vi "Init Request Poller.vi"(8 "error in (no error)":errorcluster, 10 "output_request_poller in":refnum<class "output_poller.lvclass">, 11 "output in":refnum<class "Output.lvclass">) -> (0 "error out":errorcluster, 3 "output out":refnum<class "Output.lvclass">)   [LabVIEW 2015, in "Output.lvclass"]
uses:
  Output.lvclass
  output_poller/output_poller.lvclass
  Output.lvclass/Output.ctl
  output_poller/output_poller.lvclass/output_poller.ctl
  <vilib>/ActorFramework/Actor/Actor.lvclass
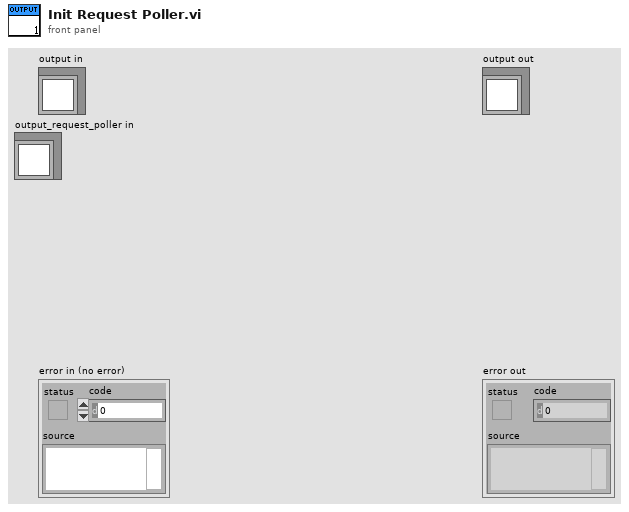
[diagram p1: front panel]
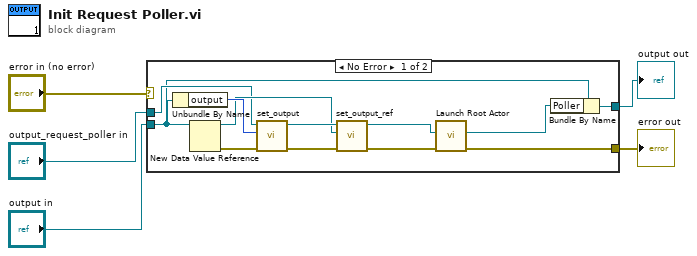
[diagram p0: block diagram]
diagram:
  n1 = case shown="No Error" "error in (no error)" {
    selector: "error in (no error)" -> [_ w19]
    tunnel: [w10 w19] -> w4
    tunnel: [w6 w18] -> w2
    tunnel: "output in" -> [w7 w18]
    tunnel: "output_request_poller in" -> [w9 _]
    frame No Error {
      n2 = Unbundle By Name(w7) -> ("output"=w16:i32)
      n3 = New Data Value Reference(data value=w7) -> (data value reference=w15:refnum<data-value>, error out=w13:errorcluster)  [unwired: 1 in]
      n4 = call "set_output.vi"("error in (no error)"=w13, "output"=w16, "output_request_poller in"=w9) -> ("error out"=w12:errorcluster, "output_request_poller out"=w17:refnum<class "output_poller.lvclass">)  [unwired: 7 in]
      n5 = call "set_output_ref.vi"("error in (no error)"=w12, "output_ref"=w15, "output_request_poller in"=w17) -> ("error out"=w11:errorcluster, "output_request_poller out"=w14:refnum<class "output_poller.lvclass">)  [unwired: 7 in]
      n6 = call <vilib>:"Launch Root Actor.vi"("error in (no error)"=w11, "Actor"=w14) -> ("error out"=w10:errorcluster, "Actor's Enqueuer"=w8:refnum<class "Message Enqueuer.lvclass">)  [unwired: 8 in]
      n7 = Bundle By Name(cluster=w7, "Poller"=w8) -> (w6:refnum<class "Output.lvclass">)
    }
    frame Error {
    }
  }
  "error out" <- w4
  "output out" <- w2
